vi "FA_MultiWriteXML.vi"(6 "Error In":errorcluster, 7 "XML String Array":string[](array[string]), 8 "Special Type Array":T1[](array[typedef])) -> (0 "Error Out":errorcluster)   [LabVIEW 2014, in "FA_LocalStore.lvlib"]
doc: "Writes an array of new XML to LocalStore for an array of Special Type."
uses:
  FA_LocalStore.lvlib
  FA_LSSpecialTypes.ctl
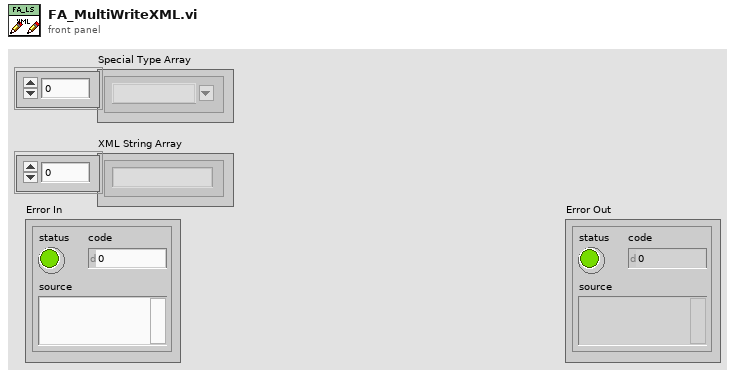
[diagram p1: front panel]
types:
  T1 = typedef "FA_LocalStore.lvlib/FA_LSSpecialTypes.ctl" = string
  T2 = typedef "FA_LocalStore.lvlib/FA_LSRef.ctl" = cluster{"eTag INI Refnum":T3, "XML Refnum Array":refnum<file>[]}
  T3 = typedef "NI_LVConfig.lvlib/Config Data RefNum.ctl" = refnum<k1>
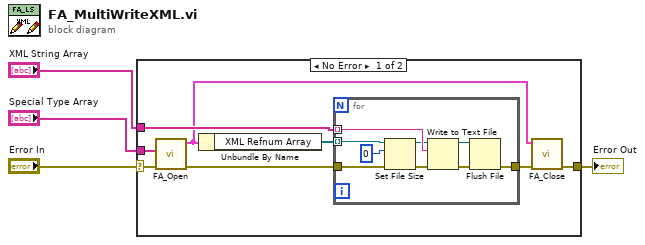
[diagram p0: block diagram]
diagram:
  n1 = case shown="No Error" "Error In" {
    selector: "Error In" -> [w9 w22]
    tunnel: [w10 w22] -> w3
    tunnel: "Special Type Array" -> [w7 _]
    tunnel: "XML String Array" -> [w12 _]
    frame No Error {
      n2 = call "FA_Open.vi"("Error In"=w9, "Special Types Array"=w7) -> ("Error Out"=w8:errorcluster, "FA_LS Ref"=w11:T2)  [unwired: 8 in]
      n3 = Unbundle By Name(w11) -> ("XML Refnum Array"=w6:refnum<file>[])
      n4 = for {
        tunnel: w12 -> [w21] mode=indexing
        tunnel: [w15] -> w5
        tunnel: w8 -> [w14]
        tunnel: w6 -> [w13] mode=indexing
        n5 = Set File Size(4:w14, 6:i64 0 ("size (in bytes)"), 7:w13) -> (0:w19:errorcluster, 3:w20:refnum<file>)
        n6 = Write to Text File(file (use dialog)=w20, text=w21, error in=w19) -> (refnum out=w16:refnum<file>, error out=w17:errorcluster)  [unwired: 1 in, 1 out]
        n7 = Flush File(refnum=w16, error in=w17) -> (error out=w15:errorcluster)  [unwired: 1 out]
      }
      n8 = call "FA_Close.vi"("Error In"=w5, "FA_LS Ref"=w11) -> ("Error Out"=w10:errorcluster)  [unwired: 9 in]
    }
    frame Error {
    }
  }
  "Error Out" <- w3
